vi "ex_ParsePacketHeader.vi"(7 "Decimal Separator":string, 8 "error in (no error)":errorcluster, 9 "file_params":T4={"include col headings?"=TRUE, "x_columns"=0, "col headings always?"=TRUE, "time preference"=0, "hide col headings"=FALSE} {"time preference" items=["Absolute", "Relative"]; "x_columns" items=["None", "One", "Multiple"]}, 10 "delimiter":string, 11 "file header string":string) -> (0 "error out":errorcluster, 1 "test info":T2, 2 "notes":string, 3 "channel info":T3[](array[typedef]) {"Delta X" format="%.2p"; "X0" format="%<%X\n%x>T"; "Timestamp" format="%<%X\n%x>T"}, 4 "UUT info":T1)   [LabVIEW 2020]
uses:
  <vilib>/express/express input/ExFileReadBlock.llb/ex_ReadFileParams.ctl
  <vilib>/express/express shared/ExFile.llb/ex_AllChanInfo.ctl
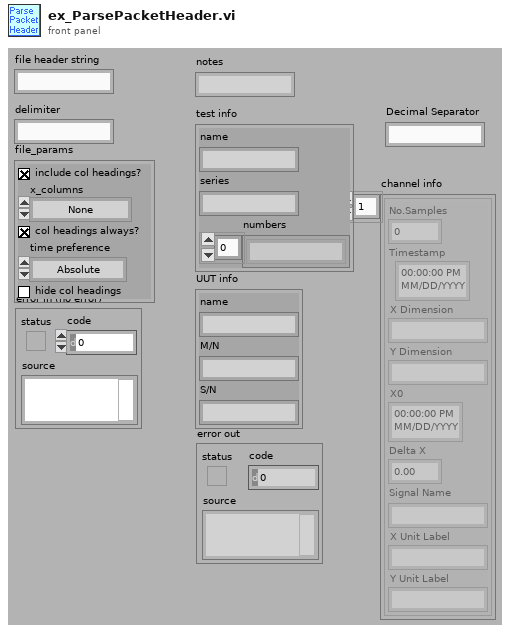
[diagram p1: front panel]
types:
  T1 = cluster{"name":string, "M/N":string, "S/N":string}
  T2 = cluster{"name":string, "series":string, "numbers":string[]}
  T3 = typedef "ex_AllChanInfo.ctl" = cluster{"No.Samples":i32, "Timestamp":timestamp, "X Dimension":string, "Y Dimension":string, "X0":timestamp, "Delta X":dbl, "Signal Name":string, "X Unit Label":string, "Y Unit Label":string}
  T4 = typedef "ex_ReadFileParams.ctl" = cluster{"include col headings?":bool, "x_columns":u16, "col headings always?":bool, "time preference":u16, "hide col headings":bool}
  T5 = cluster{"UUTName":string, "UUTM/N":string, "UUTS/N":string}
  T6 = cluster{"TestName":string, "TestSeries":string, "TestNumbers":string[]}
  T7 = cluster{"Date":bool, "Time":bool, "X0":bool, "DeltaX":bool, "Samples":bool, "XDimension":bool, "XUnitLabel":bool, "YDimension":bool, "YUnitLabel":bool}
  T8 = cluster{"Date":string, "Time":string, "Notes":string, "TestName":string, "TestNumbers":string[], "TestSeries":string, "UUTM/N":string, "UUTName":string, "UUTS/N":string, "XDimension":string, "XUnitLabel":string, "YDimension":string, "YUnitLabel":string}
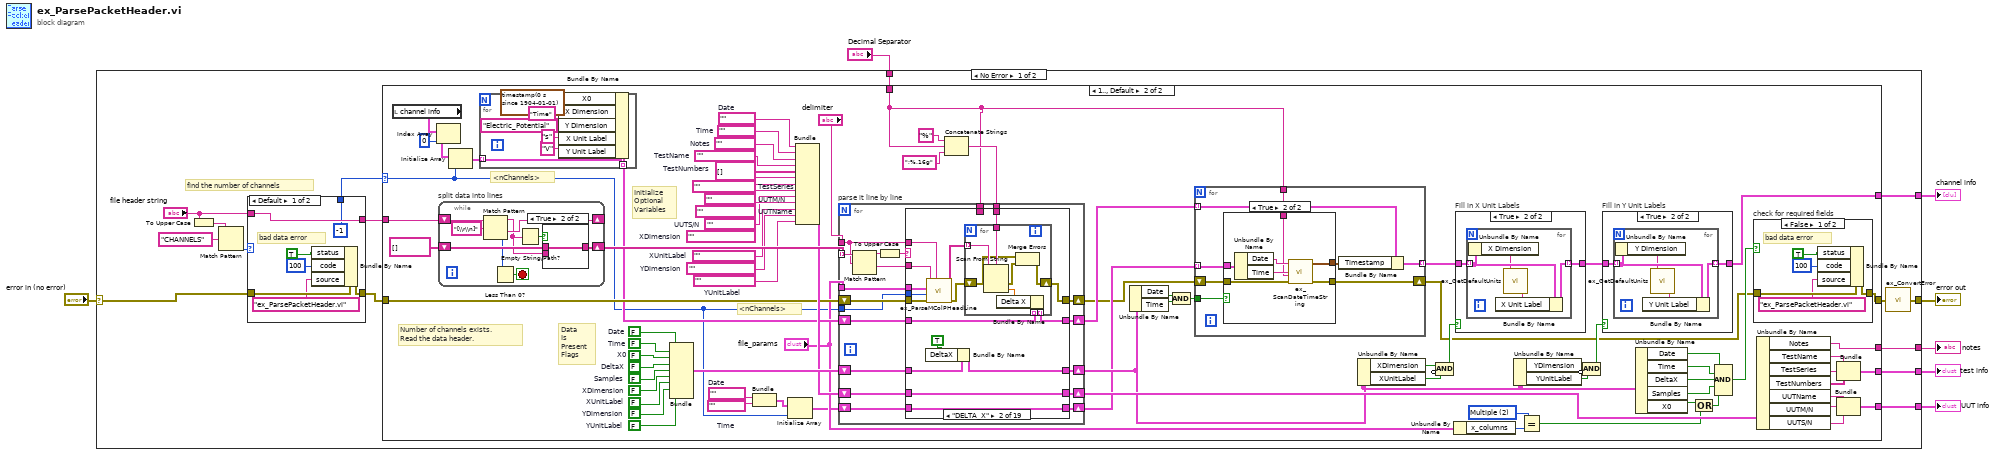
[diagram p0: block diagram]
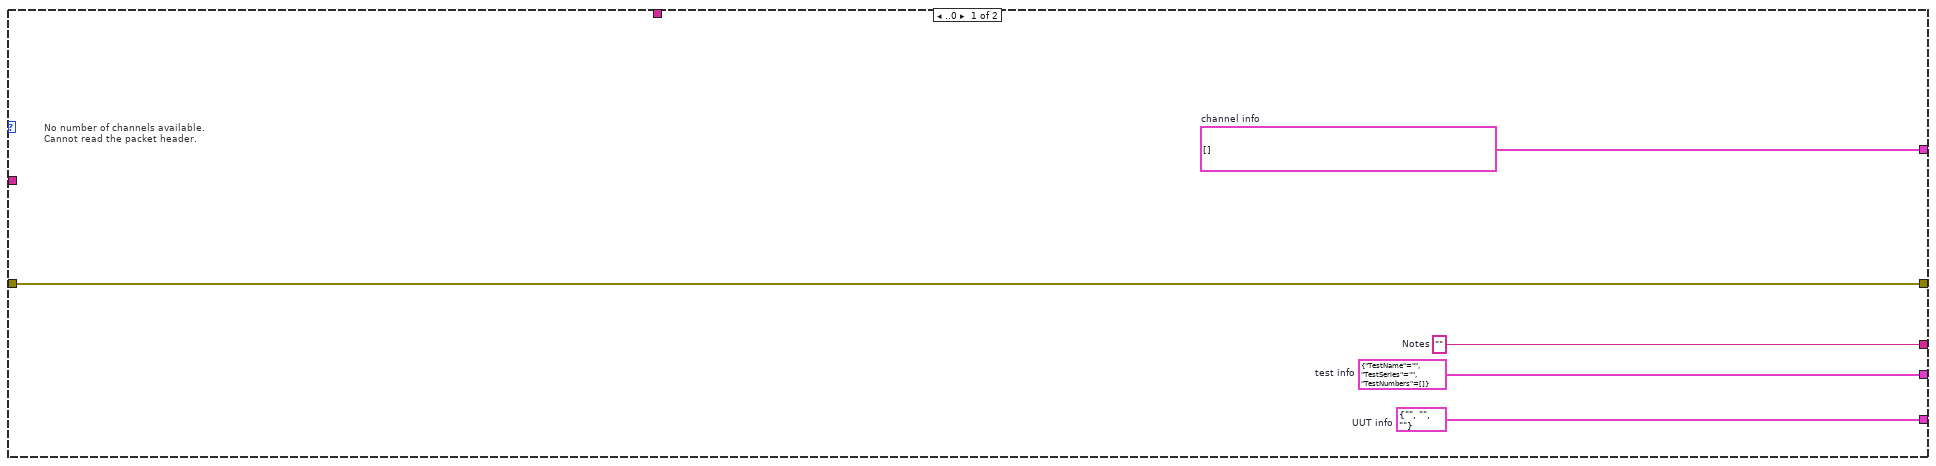
[diagram p2: hidden frame]
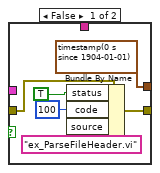
[diagram p3: hidden frame]
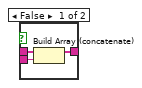
[diagram p7: hidden frame]
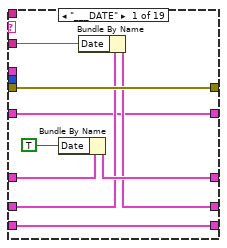
[diagram p8: hidden frame]
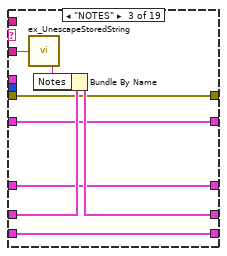
[diagram p9: hidden frame]
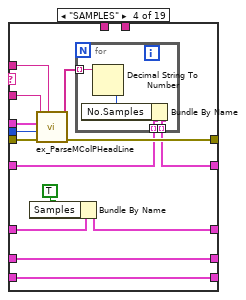
[diagram p10: hidden frame]
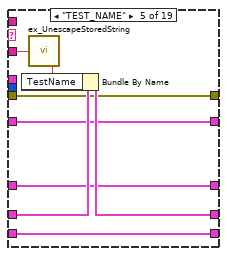
[diagram p11: hidden frame]
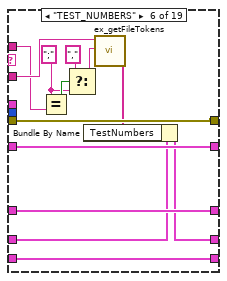
[diagram p12: hidden frame]
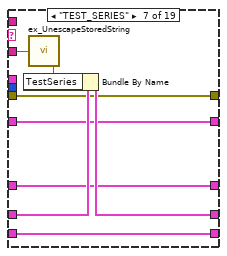
[diagram p13: hidden frame]
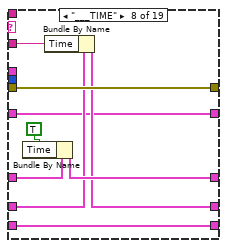
[diagram p14: hidden frame]
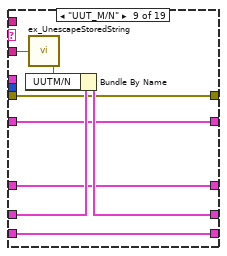
[diagram p15: hidden frame]
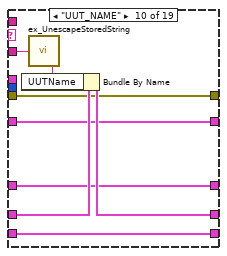
[diagram p16: hidden frame]
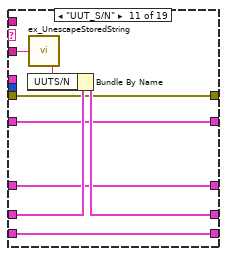
[diagram p17: hidden frame]
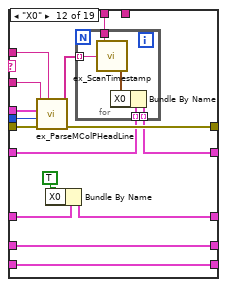
[diagram p18: hidden frame]
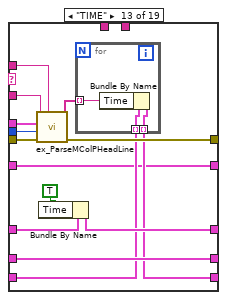
[diagram p19: hidden frame]
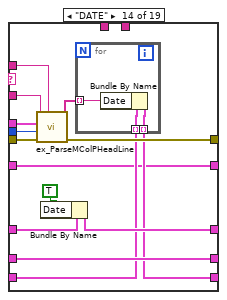
[diagram p20: hidden frame]
diagram:
  n1 = case shown="No Error" "error in (no error)" {
    selector: "error in (no error)" -> [w17 w461]
    tunnel: [w18 w461] -> w6
    tunnel: [w13 T3[] []] -> w5
    tunnel: [w12 ""] -> w4
    tunnel: [w11 T6 {"TestName"="", "TestSeries"="", "TestNumbers"=[]}] -> w3
    tunnel: [w10 T5 {"UUTName"="", "UUTM/N"="", "UUTS/N"=""}] -> w2
    tunnel: "Decimal Separator" -> [w8 _]
    frame No Error {
      # "find the number of channels"
      n2 = To Upper Case(1:"file header string") -> (0:w21:string)
      n3 = Match Pattern(string=w21, regular expression="CHANNELS") -> (offset past match=w20:i32)  [unwired: 4 out]
      n4 = case shown="Default" w20 {
        selector: w20 -> [_ w454]
        tunnel: "file header string" -> [w448 w455]
        tunnel: [w448 w455] -> w16
        tunnel: w17 -> [w447 w450]
        tunnel: [w446 w450] -> w15
        tunnel: [-1 w449] -> w9
        frame Default {
          # "bad data error"
          n5 = Bundle By Name(cluster=w447, "status"=TRUE, "code"=100, "source"="ex_ParsePacketHeader.vi") -> (w446:errorcluster)
        }
        frame 0.. {
          n6 = Increment(x=w454) -> (x+1=w452:i32)
          n7 = Match Pattern(string=w455, regular expression="[\\r\\n]", offset (0)=w454) -> (before substring=w453:string)  [unwired: 3 out]
          n8 = Decimal String To Number(string=w453, offset=w452, default (0L)=0) -> (number=w449:i32)  [unwired: 1 out]
        }
      }
      n9 = case shown="1.., Default" w9 {
        selector: w9 -> [_ w32]
        tunnel: w16 -> [_ w95]
        tunnel: w15 -> [w27 w93]
        tunnel: [w27 w61] -> w14
        tunnel: [w26 w60] -> w13
        tunnel: [w25 w56] -> w12
        tunnel: [w24 w53] -> w11
        tunnel: [w23 w48] -> w10
        tunnel: w8 -> [_ w28]
        frame ..0 {
          w23 = T5 {"UUTName"="", "UUTM/N"="", "UUTS/N"=""}  # UUT info
          w24 = T6 {"TestName"="", "TestSeries"="", "TestNumbers"=[]}  # test info
          w26 = T3[] []  # channel info
          w25 = ""  # Notes
          # "No number of channels available.\nCannot read the packet header."
        }
        frame 1.., Default {
          w43 = u16 2 items=["None", "One", "Multiple"] ("x_columns")
          w39 = ""  # Time
          w40 = ""  # Date
          w86 = ""  # Time
          w87 = ""  # Date
          w88 = ""  # YUnitLabel
          w82 = ""  # YDimension
          w81 = ""  # XUnitLabel
          w80 = ""  # XDimension
          w79 = ""  # UUTS/N
          w78 = ""  # UUTName
          w83 = string[] []  # TestNumbers
          w97 = FALSE  # XDimension
          w98 = FALSE  # XUnitLabel
          w99 = FALSE  # YDimension
          w100 = FALSE  # YUnitLabel
          w96 = FALSE  # Samples
          w77 = ""  # UUTM/N
          w76 = ""  # TestSeries
          w103 = FALSE  # DeltaX
          w84 = ""  # TestName
          w85 = ""  # Notes
          w107 = FALSE  # X0
          w109 = FALSE  # Time
          w108 = FALSE  # Date
          # "Number of channels exists.\nRead the data header."
          # "<nChannels>"
          # "Initialize\nOptional\nVariables"
          # "<nChannels>"
          # "Data\nIs\nPresent\nFlags"
          n10 = local read "channel info"() -> (w92:T3[])
          n11 = Index Array(array=w92, index=0) -> (element=w90:T3)
          n12 = while "split data into lines" {
            shift-right: [w160] -> _
            shift-left: w95 -> [w166]
            shift-right: [w164] -> w105
            shift-left: string[] [] -> [w165]
            stop <- w162 stop-if-true
            n13 = Match Pattern(string=w166, regular expression="[\\r\\n]") -> (before substring=w159:string, after substring=w160:string, offset past match=w163:i32)  [unwired: 2 out]
            n14 = Less Than 0?(x=w163) -> (x < 0?=w162:bool)
            n15 = Empty String/Path?(string/path=w159) -> (empty?=w158:bool)
            n16 = case shown="True" w158 {
              tunnel: w165 -> [w169 w170]
              tunnel: w159 -> [w168 _]
              tunnel: [w167 w170] -> w164
              frame False {
                n17 = Build Array (concatenate)(w169, w168) -> (w167:string[])
              }
              frame True {
              }
            }
          }
          n18 = Initialize Array(w90, w32) -> (w89:T3[])
          n19 = for {
            tunnel: w89 -> [w157] mode=indexing
            tunnel: [w152] -> w74 mode=indexing
            n20 = Bundle By Name(cluster=w157, "X0"=timestamp(0 s since 1904-01-01), "X Dimension"="Time", "Y Dimension"="Electric_Potential", "X Unit Label"="s", "Y Unit Label"="V") -> (w152:T3)
          }
          n21 = Bundle("Date"=w108, "Time"=w109, "X0"=w107, "DeltaX"=w103, "Samples"=w96, "XDimension"=w97, "XUnitLabel"=w98, "YDimension"=w99, "YUnitLabel"=w100) -> (w106:T7)  [unwired: 1 out]
          n22 = Bundle("Date"=w40, "Time"=w39) -> (w38:cluster{"Date":string, "Time":string})  [unwired: 1 out]
          n23 = Initialize Array(w38, w32) -> (w37:cluster{"Date":string, "Time":string}[])
          n24 = Bundle("Date"=w87, "Time"=w86, "Notes"=w85, "TestName"=w84, "TestNumbers"=w83, "TestSeries"=w76, "UUTM/N"=w77, "UUTName"=w78, "UUTS/N"=w79, "XDimension"=w80, "XUnitLabel"=w81, "YDimension"=w82, "YUnitLabel"=w88) -> (w104:T8)  [unwired: 1 out]
          n25 = Concatenate Strings("%" ("string"), w28, ";%.16g" ("string")) -> (w29:string)
          n26 = for "parse it line by line" {
            tunnel: w105 -> [w189] mode=indexing
            tunnel: "delimiter" -> [w179]
            shift-right: [w184] -> w35
            shift-left: w93 -> [w185]
            shift-right: [w181] -> w41
            shift-left: w106 -> [w183]
            shift-right: [w180] -> w59
            shift-left: w104 -> [w182]
            tunnel: w32 -> [w178]
            shift-right: [w176] -> w58
            shift-left: w74 -> [w177]
            tunnel: "file_params" -> [w175]
            shift-right: [w173] -> w36
            shift-left: w37 -> [w174]
            tunnel: w29 -> [w172]
            tunnel: w28 -> [w171]
            n27 = Match Pattern(string=w189, regular expression=w179) -> (before substring=w188:string, after substring=w186:string)  [unwired: 3 out]
            n28 = To Upper Case(1:w188) -> (0:w187:string)
            n29 = case shown="\"DELTA_X\"" w187 {
              tunnel: w186 -> [w193 w213 w230 w243 w256 w265 w277 w279 w294 w302 w310 w324 w343 w360 w377 w395 w413 w431 _]
              tunnel: w185 -> [w198 w214 w224 w244 w250 w263 w271 w283 w288 w296 w304 w325 w344 w361 w378 w396 w414 w432 w441]
              tunnel: [w198 w201 w224 w236 w250 w263 w271 w283 w288 w296 w304 w317 w336 w353 w370 w388 w406 w424 w441] -> w184
              tunnel: w183 -> [w197 w209 w226 w239 w252 w261 w273 w286 w290 w298 w306 w320 w339 w356 w373 w391 w409 w427 w440]
              tunnel: w182 -> [w194 w203 w229 w232 w255 w260 w276 w282 w293 w301 w309 w313 w334 w351 w366 w384 w402 w420 w439]
              tunnel: [w195 w207 w226 w237 w252 w261 w273 w285 w290 w298 w306 w318 w337 w354 w371 w389 w407 w425 w440] -> w181
              tunnel: [w192 w203 w227 w232 w253 w258 w274 w281 w291 w299 w307 w313 w334 w351 w366 w384 w402 w420 w439] -> w180
              tunnel: w179 -> [_ w212 _ w242 _ w264 _ _ _ _ _ w323 w342 w359 w376 w394 w412 w430 _]
              tunnel: w175 -> [_ w211 _ w241 _ _ _ _ _ _ _ w322 w341 w358 w375 w393 w411 w429 _]
              tunnel: w178 -> [_ w210 _ w240 _ _ _ _ _ _ _ w321 w340 w357 w374 w392 w410 w428 _]
              tunnel: w177 -> [w191 w205 w225 w234 w251 w262 w272 w280 w289 w297 w305 w315 w331 w348 w368 w386 w404 w422 w438]
              tunnel: [w191 w204 w225 w233 w251 w262 w272 w280 w289 w297 w305 w314 w331 w348 w367 w385 w403 w421 w438] -> w176
              tunnel: w174 -> [w190 w200 w223 w231 w249 w257 w270 w278 w287 w295 w303 w312 w333 w350 w365 w383 w401 w419 w437]
              tunnel: [w190 w200 w223 w231 w249 w257 w270 w278 w287 w295 w303 w312 w332 w349 w365 w383 w401 w419 w437] -> w173
              tunnel: w172 -> [_ w199 _ _ _ _ _ _ _ _ _ _ _ _ _ _ _ _ _]
              tunnel: w171 -> [_ _ _ _ _ _ _ _ _ _ _ w311 _ _ _ _ _ _ _]
              frame "___DATE" {
                n30 = Bundle By Name(cluster=w197, "Date"=TRUE ("Date?")) -> (w195:T7)
                n31 = Bundle By Name(cluster=w194, "Date"=w193) -> (w192:T8)
              }
              frame "DELTA_X" {
                n32 = Bundle By Name(cluster=w209, "DeltaX"=TRUE) -> (w207:T7)
                n33 = call <vilib>:"ex_ParseMColPHeadLine.vi"("delimiter"=w212, "error in (no error)"=w214, "channels"=w210, "file_params"=w211, "line"=w213) -> ("error out"=w202:errorcluster, "elements"=w206:string[])  [unwired: 5 out]
                n34 = for {
                  tunnel: w206 -> [w220] mode=indexing
                  tunnel: w205 -> [w222] mode=indexing
                  tunnel: [w221] -> w204 mode=indexing
                  shift-right: [w215] -> w201
                  shift-left: w202 -> [w217]
                  tunnel: w199 -> [w219]
                  n35 = Scan From String(format string=w219, input string=w220) -> (error out=w216:errorcluster, output 1=w218:dbl)  [unwired: 2 in, 3 out]
                  n36 = Bundle By Name(cluster=w222, "Delta X"=w218) -> (w221:T3)
                  n37 = Merge Errors(w217, w216) -> (w215:errorcluster)
                }
              }
              frame "NOTES" {
                n38 = call <vilib>:"ex_UnescapeStoredString.vi"("stored string"=w230) -> ("parsed string"=w228:string)
                n39 = Bundle By Name(cluster=w229, "Notes"=w228) -> (w227:T8)
              }
              frame "SAMPLES" {
                n40 = Bundle By Name(cluster=w239, "Samples"=TRUE ("DeltaX")) -> (w237:T7)
                n41 = call <vilib>:"ex_ParseMColPHeadLine.vi"("delimiter"=w242, "error in (no error)"=w244, "channels"=w240, "file_params"=w241, "line"=w243) -> ("error out"=w236:errorcluster, "elements"=w235:string[])  [unwired: 5 out]
                n42 = for {
                  tunnel: w235 -> [w248] mode=indexing
                  tunnel: w234 -> [w247] mode=indexing
                  tunnel: [w246] -> w233 mode=indexing
                  n43 = Decimal String To Number(string=w248) -> (number=w245:i32)  [unwired: 3 out]
                  n44 = Bundle By Name(cluster=w247, "No.Samples"=w245) -> (w246:T3)
                }
              }
              frame "TEST_NAME" {
                n45 = call <vilib>:"ex_UnescapeStoredString.vi"("stored string"=w256) -> ("parsed string"=w254:string)
                n46 = Bundle By Name(cluster=w255, "TestName"=w254) -> (w253:T8)
              }
              frame "TEST_NUMBERS" {
                w268 = ";"
                n47 = Equal?(x=w268, y=w264) -> (x = y?=w269:bool)
                n48 = Select(t=",", s=w269, f=w268) -> (s? t:f=w266:string)
                n49 = call <vilib>:"ex_getFileTokens.vi"("delimiters"=w266, "delimited string"=w265) -> ("tokens"=w259:string[])  [unwired: 7 out]
                n50 = Bundle By Name(cluster=w260, "TestNumbers"=w259) -> (w258:T8)
              }
              frame "TEST_SERIES" {
                n51 = call <vilib>:"ex_UnescapeStoredString.vi"("stored string"=w277) -> ("parsed string"=w275:string)
                n52 = Bundle By Name(cluster=w276, "TestSeries"=w275) -> (w274:T8)
              }
              frame "___TIME" {
                n53 = Bundle By Name(cluster=w286, "Time"=TRUE ("Time?")) -> (w285:T7)
                n54 = Bundle By Name(cluster=w282, "Time"=w279) -> (w281:T8)
              }
              frame "UUT_M/N" {
                n55 = call <vilib>:"ex_UnescapeStoredString.vi"("stored string"=w294) -> ("parsed string"=w292:string)
                n56 = Bundle By Name(cluster=w293, "UUTM/N"=w292) -> (w291:T8)
              }
              frame "UUT_NAME" {
                n57 = call <vilib>:"ex_UnescapeStoredString.vi"("stored string"=w302) -> ("parsed string"=w300:string)
                n58 = Bundle By Name(cluster=w301, "UUTName"=w300) -> (w299:T8)
              }
              frame "UUT_S/N" {
                n59 = call <vilib>:"ex_UnescapeStoredString.vi"("stored string"=w310) -> ("parsed string"=w308:string)
                n60 = Bundle By Name(cluster=w309, "UUTS/N"=w308) -> (w307:T8)
              }
              frame "X0" {
                n61 = call <vilib>:"ex_ParseMColPHeadLine.vi"("delimiter"=w323, "error in (no error)"=w325, "channels"=w321, "file_params"=w322, "line"=w324) -> ("error out"=w317:errorcluster, "elements"=w316:string[])  [unwired: 5 out]
                n62 = Bundle By Name(cluster=w320, "X0"=TRUE ("DeltaX")) -> (w318:T7)
                n63 = for {
                  tunnel: w316 -> [w328] mode=indexing
                  tunnel: w315 -> [w330] mode=indexing
                  tunnel: [w329] -> w314 mode=indexing
                  tunnel: w311 -> [w326]
                  n64 = call <vilib>:"ex_ScanTimestamp.vi"("High-Precision Numeric String"=w328, "Decimal point"=w326) -> ("High-Precision Numeric"=w327:timestamp)  [unwired: 1 in, 2 out]
                  n65 = Bundle By Name(cluster=w330, "X0"=w327) -> (w329:T3)
                }
              }
              frame "TIME" {
                n66 = call <vilib>:"ex_ParseMColPHeadLine.vi"("delimiter"=w342, "error in (no error)"=w344, "channels"=w340, "file_params"=w341, "line"=w343) -> ("error out"=w336:errorcluster, "elements"=w335:string[])  [unwired: 5 out]
                n67 = Bundle By Name(cluster=w339, "Time"=TRUE ("DeltaX")) -> (w337:T7)
                n68 = for {
                  tunnel: w335 -> [w345] mode=indexing
                  tunnel: w333 -> [w347] mode=indexing
                  tunnel: [w346] -> w332 mode=indexing
                  n69 = Bundle By Name(cluster=w347, "Time"=w345) -> (w346:cluster{"Date":string, "Time":string})
                }
              }
              frame "DATE" {
                n70 = call <vilib>:"ex_ParseMColPHeadLine.vi"("delimiter"=w359, "error in (no error)"=w361, "channels"=w357, "file_params"=w358, "line"=w360) -> ("error out"=w353:errorcluster, "elements"=w352:string[])  [unwired: 5 out]
                n71 = Bundle By Name(cluster=w356, "Date"=TRUE ("DeltaX")) -> (w354:T7)
                n72 = for {
                  tunnel: w352 -> [w362] mode=indexing
                  tunnel: w350 -> [w364] mode=indexing
                  tunnel: [w363] -> w349 mode=indexing
                  n73 = Bundle By Name(cluster=w364, "Date"=w362) -> (w363:cluster{"Date":string, "Time":string})
                }
              }
              frame "X_DIMENSION" {
                n74 = Bundle By Name(cluster=w373, "XDimension"=TRUE ("DeltaX")) -> (w371:T7)
                n75 = call <vilib>:"ex_ParseMColPHeadLine.vi"("delimiter"=w376, "error in (no error)"=w378, "channels"=w374, "file_params"=w375, "line"=w377) -> ("error out"=w370:errorcluster, "elements"=w369:string[])  [unwired: 5 out]
                n76 = for {
                  tunnel: w369 -> [w379] mode=indexing
                  tunnel: w368 -> [w382] mode=indexing
                  tunnel: [w381] -> w367 mode=indexing
                  n77 = call <vilib>:"ex_UnescapeStoredString.vi"("stored string"=w379) -> ("parsed string"=w380:string)
                  n78 = Bundle By Name(cluster=w382, "X Dimension"=w380) -> (w381:T3)
                }
              }
              frame "X_UNIT_LABEL" {
                n79 = Bundle By Name(cluster=w391, "XUnitLabel"=TRUE ("DeltaX")) -> (w389:T7)
                n80 = call <vilib>:"ex_ParseMColPHeadLine.vi"("delimiter"=w394, "error in (no error)"=w396, "channels"=w392, "file_params"=w393, "line"=w395) -> ("error out"=w388:errorcluster, "elements"=w387:string[])  [unwired: 5 out]
                n81 = for {
                  tunnel: w387 -> [w397] mode=indexing
                  tunnel: w386 -> [w400] mode=indexing
                  tunnel: [w399] -> w385 mode=indexing
                  n82 = call <vilib>:"ex_UnescapeStoredString.vi"("stored string"=w397) -> ("parsed string"=w398:string)
                  n83 = Bundle By Name(cluster=w400, "X Unit Label"=w398) -> (w399:T3)
                }
              }
              frame "Y_DIMENSION" {
                n84 = Bundle By Name(cluster=w409, "YDimension"=TRUE ("DeltaX")) -> (w407:T7)
                n85 = call <vilib>:"ex_ParseMColPHeadLine.vi"("delimiter"=w412, "error in (no error)"=w414, "channels"=w410, "file_params"=w411, "line"=w413) -> ("error out"=w406:errorcluster, "elements"=w405:string[])  [unwired: 5 out]
                n86 = for {
                  tunnel: w405 -> [w415] mode=indexing
                  tunnel: w404 -> [w418] mode=indexing
                  tunnel: [w417] -> w403 mode=indexing
                  n87 = call <vilib>:"ex_UnescapeStoredString.vi"("stored string"=w415) -> ("parsed string"=w416:string)
                  n88 = Bundle By Name(cluster=w418, "Y Dimension"=w416) -> (w417:T3)
                }
              }
              frame "Y_UNIT_LABEL" {
                n89 = Bundle By Name(cluster=w427, "YUnitLabel"=TRUE ("DeltaX")) -> (w425:T7)
                n90 = call <vilib>:"ex_ParseMColPHeadLine.vi"("delimiter"=w430, "error in (no error)"=w432, "channels"=w428, "file_params"=w429, "line"=w431) -> ("error out"=w424:errorcluster, "elements"=w423:string[])  [unwired: 5 out]
                n91 = for {
                  tunnel: w423 -> [w433] mode=indexing
                  tunnel: w422 -> [w436] mode=indexing
                  tunnel: [w435] -> w421 mode=indexing
                  n92 = call <vilib>:"ex_UnescapeStoredString.vi"("stored string"=w433) -> ("parsed string"=w434:string)
                  n93 = Bundle By Name(cluster=w436, "Y Unit Label"=w434) -> (w435:T3)
                }
              }
              frame Default {
              }
            }
          }
          n94 = Unbundle By Name(w41) -> ("Date"=w101:bool, "Time"=w102:bool)
          n95 = And(x=w101, y=w102) -> (x .and. y?=w33:bool)
          n96 = for {
            tunnel: w58 -> [w117] mode=indexing
            tunnel: [w116] -> w57 mode=indexing
            tunnel: w36 -> [w114] mode=indexing
            shift-right: [w112] -> w34
            shift-left: w35 -> [w113]
            tunnel: w33 -> [w111]
            tunnel: w28 -> [w110]
            n97 = case shown="True" w111 {
              tunnel: [timestamp(0 s since 1904-01-01) w130] -> w115
              tunnel: w114 -> [_ w127]
              tunnel: w113 -> [w118 w126]
              tunnel: [w119 w125] -> w112
              tunnel: w110 -> [_ w124]
              frame False {
                n98 = Bundle By Name(cluster=w118, "status"=TRUE, "code"=100, "source"="ex_ParseFileHeader.vi") -> (w119:errorcluster)
              }
              frame True {
                n99 = Unbundle By Name(w127) -> ("Date"=w129:string, "Time"=w128:string)
                n100 = call <vilib>:"ex_ScanDateTimeString.vi"("error in (no error)"=w126, "Decimal point"=w124, "Time String"=w128, "Date String"=w129) -> ("error out"=w125:errorcluster, "Date/Time in seconds"=w130:timestamp)  [unwired: 2 out]
              }
            }
            n101 = Bundle By Name(cluster=w117, "Timestamp"=w115) -> (w116:T3)
          }
          n102 = Unbundle By Name(w41) -> ("XDimension"=w72:bool, "XUnitLabel"=w73:bool)
          n103 = Compound Arithmetic op=AND(w72, invert w73) -> (w71:bool)
          n104 = Unbundle By Name("file_params") -> ("x_columns"=w42:u16)
          n105 = case "Fill in X Unit Labels" shown="True" w71 {
            tunnel: w57 -> [w144 w146]
            tunnel: [w144 w145] -> w67
            frame False {
            }
            frame True {
              n106 = for {
                tunnel: w146 -> [w150] mode=indexing
                tunnel: [w147] -> w145 mode=indexing
                n107 = Unbundle By Name(w150) -> ("X Dimension"=w149:string)
                n108 = call <vilib>:"ex_GetDefaultUnits.vi"("dimension"=w149) -> ("default units"=w148:string)
                n109 = Bundle By Name(cluster=w150, "X Unit Label"=w148) -> (w147:T3)
              }
            }
          }
          n110 = Unbundle By Name(w41) -> ("YDimension"=w69:bool, "YUnitLabel"=w68:bool)
          n111 = Equal?(x=w43, y=w42) -> (x = y?=w44:bool)
          n112 = Compound Arithmetic op=AND(w69, invert w68) -> (w70:bool)
          n113 = case "Fill in Y Unit Labels" shown="True" w70 {
            tunnel: w67 -> [w137 w139]
            tunnel: [w137 w138] -> w60
            frame False {
            }
            frame True {
              n114 = for {
                tunnel: w139 -> [w143] mode=indexing
                tunnel: [w140] -> w138 mode=indexing
                n115 = Unbundle By Name(w143) -> ("Y Dimension"=w142:string)
                n116 = call <vilib>:"ex_GetDefaultUnits.vi"("dimension"=w142) -> ("default units"=w141:string)
                n117 = Bundle By Name(cluster=w143, "Y Unit Label"=w141) -> (w140:T3)
              }
            }
          }
          n118 = Unbundle By Name(w41) -> ("Date"=w66:bool, "Time"=w64:bool, "DeltaX"=w65:bool, "Samples"=w63:bool, "X0"=w45:bool)
          n119 = Or(x=w45, y=w44) -> (x .or. y?=w46:bool)
          n120 = Compound Arithmetic op=AND(w66, w64, w65, w63, w46) -> (w62:bool)
          n121 = case "check for required fields" shown="False" w62 {
            tunnel: w34 -> [w135 w136]
            tunnel: [w134 w136] -> w61
            frame False {
              # "bad data error"
              n122 = Bundle By Name(cluster=w135, "status"=TRUE, "code"=100, "source"="ex_ParsePacketHeader.vi") -> (w134:errorcluster)
            }
            frame True {
            }
          }
          n123 = Unbundle By Name(w59) -> ("Notes"=w56:string, "TestName"=w54:string, "TestSeries"=w55:string, "TestNumbers"=w52:string[], "UUTName"=w50:string, "UUTM/N"=w51:string, "UUTS/N"=w49:string)
          n124 = Bundle("TestName"=w54, "TestSeries"=w55, "TestNumbers"=w52) -> (w53:T6)  [unwired: 1 out]
          n125 = Bundle("UUTName"=w50, "UUTM/N"=w51, "UUTS/N"=w49) -> (w48:T5)  [unwired: 1 out]
        }
      }
      n126 = call <vilib>:"ex_ConvertError.vi"("error in (no error)"=w14) -> ("error out"=w18:errorcluster)  [unwired: 4 out]
    }
    frame Error {
    }
  }
  "error out" <- w6
  "UUT info" <- w2
  "notes" <- w4
  "test info" <- w3
  "channel info" <- w5
